vi "Decode.vi"(10 "Wire Type":T2, 11 "Buffer":u8[](array[numeric]) format="%.0x") -> (2 "error out":errorcluster, 3 "Command Data":T1 {"Time Stamp" format="%<%x %.3X>T"})   [LabVIEW 2023, in "ConstellationCommand.lvlib"]
uses:
  ConstellationCommand.lvlib
  <vilib>/IlluminatedG/IG Protoc/LV-Proto/Wire Type.ctl
  <vilib>/IlluminatedG/IG Protoc/LV-Proto/LV-Proto.lvlib
  Data.ctl
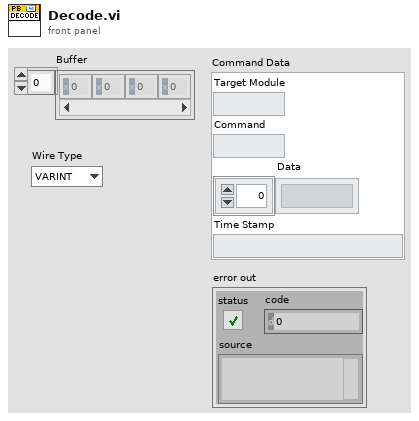
[diagram p1: front panel]
types:
  T1 = typedef "ConstellationCommand.lvlib/Data.ctl" = cluster{"Target Module":string, "Command":string, "Data":string[], "Time Stamp":timestamp}
  T2 = typedef "LV-Proto.lvlib/Wire Type.ctl" = enum8{"VARINT", "I64", "LEN", "SGROUP (Deprecated)", "EGROUP (Deprecated)", "I32"}
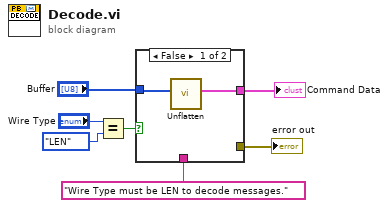
[diagram p0: block diagram]
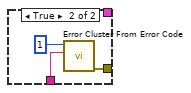
[diagram p2: hidden frame]
diagram:
  n1 = Equal?(x="Wire Type", y=Wire_Type."LEN") -> (x = y?=w2:bool)
  n2 = case shown="False" w2 {
    tunnel: "Wire Type must be LEN to decode messages." -> [_ w11]
    tunnel: [_ w10] -> w4
    tunnel: "Buffer" -> [w9 _]
    tunnel: [w8 _] -> w1
    frame False {
      n3 = call "Unflatten.vi"("Buffer"=w9) -> ("Command Data"=w8:T1)  [unwired: 9 in, 1 out]
    }
    frame True {
      n4 = call <vilib>:"Error Cluster From Error Code.vi"("error message (\"\")"=w11, "error code (0)"=1) -> ("error out"=w10:errorcluster)  [unwired: 7 in]
    }
  }
  "error out" <- w4
  "Command Data" <- w1
